vi "joystick deadband.vi"(4 "Joystick In":dbl) -> (1 "Output":dbl)   [LabVIEW 2011]
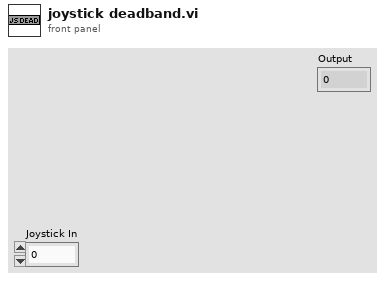
[diagram p1: front panel]
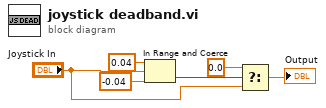
[diagram p0: block diagram]
diagram:
  n1 = In Range and Coerce(upper limit=0.04, x="Joystick In", lower limit=-0.04) -> (In Range?=w4:bool)  [unwired: 1 out]
  n2 = Select(t=0.0, s=w4, f="Joystick In") -> (s? t:f=→"Output":dbl)
